vi "Stop Controller.vi"(8 "error in (no error)":errorcluster, 11 "TestStand Controller Queue":refnum<class "Message Enqueuer.lvclass">) -> (0 "error out":errorcluster)   [LabVIEW 2015, in "TestStand API.lvlib"]
uses:
  TestStand API.lvlib
  <vilib>/ActorFramework/Message Enqueuer/Message Enqueuer.lvclass
  <userlib>/Measurement Utility API/Controller API.lvclass
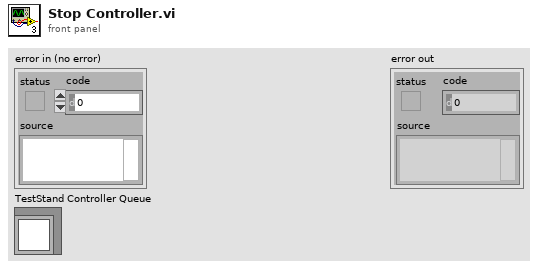
[diagram p1: front panel]
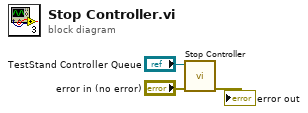
[diagram p0: block diagram]
diagram:
  n1 = call <userlib>:"Stop Controller.vi"("error in (no error)"="error in (no error)", "TestStand Controller Queue"="TestStand Controller Queue") -> ("error out"=→"error out":errorcluster)  [unwired: 9 in]
